vi "User Console.vi"(8 "error in":errorcluster) -> (0 "error out":errorcluster)   [LabVIEW 2025, in "Simulated Console.lvlib"]
doc: "This is the top level of the simulated console module (a free running module of the ATM simulator). \n\nIt is closed using a user event or a local Stop button. It communicates with the other modules using a\nqueue based API which has comms modules that can be swapped if required."
uses:
  Simulated Console.lvlib
  User Events/Controls/UE Abort Action.ctl
  Private Controls/Module Action.ctl
  Private Controls/Module Data Cluster.ctl
  Error Handler/Error Handler.lvlib
  Controller/Contoller.lvlib
  Display/Display Console/Display Console.lvlib
  Private Controls/keypad.ctl
panel:
  in  "Transactions":T1
  in  "Keypad":T2
  in  "Card Reader":bool
  # "[Covers: UI1]"
  # "[Covers: UI2]"
  # "[Covers: UI2A]"
  # "[Covers: UI2B]"
  # "[Covers: UI2C]"
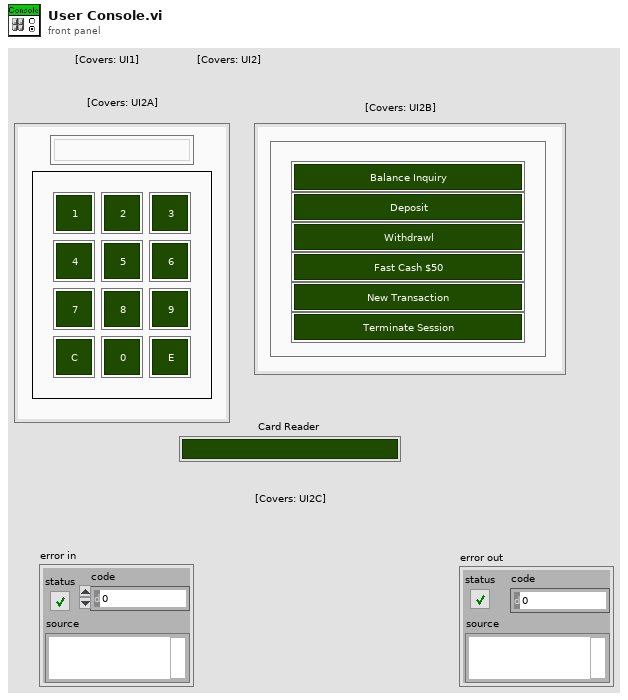
[diagram p1: front panel]
types:
  T1 = cluster{"xaction":bool, "xaction 2":bool, "xaction 3":bool, "xaction 4":bool, "xaction 5":bool, "xaction 6":bool}
  T2 = typedef "Simulated Console.lvlib/keypad.ctl" = cluster{"Key":bool, "Key 2":bool, "Key 3":bool, "Key 4":bool, "Key 5":bool, "Key 6":bool, "Key 7":bool, "Key 8":bool, "Key 9":bool, "Key 10":bool, "Key 11":bool, "Key 12":bool, "Knumber":string}
  T3 = typedef "Simulated Console.lvlib/Module Data Cluster.ctl" = cluster{"Data":variant, "Action":T4}
  T4 = typedef "Simulated Console.lvlib/Module Action.ctl" = enum16{"Error", "Init", "Card", "CancelTransaction", "NewTransaction", "Transaction", "Keypad", "Idle"}
  T5 = typedef "UE Abort Action.ctl" = enum16{"Destroy", "Get", "Create"}
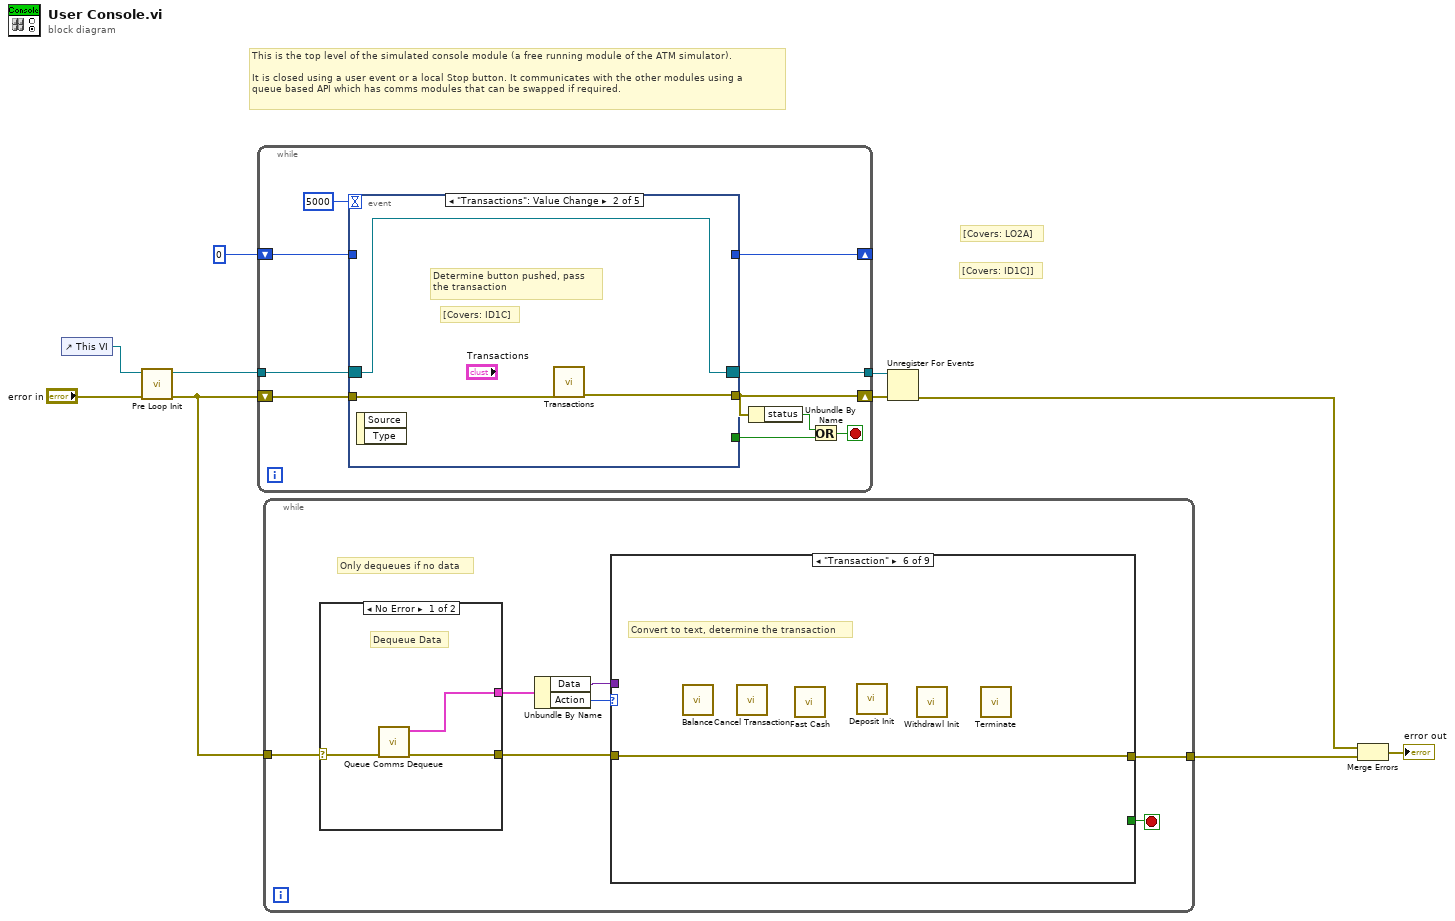
[diagram p0: block diagram]
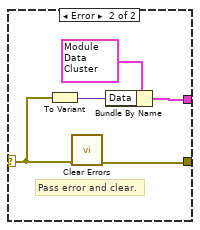
[diagram p2: hidden frame]
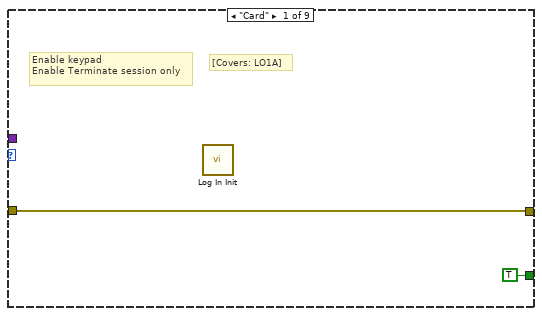
[diagram p3: hidden frame]
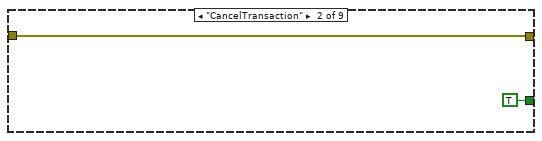
[diagram p4: hidden frame]
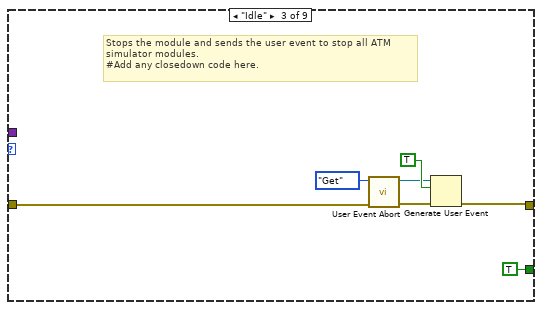
[diagram p5: hidden frame]
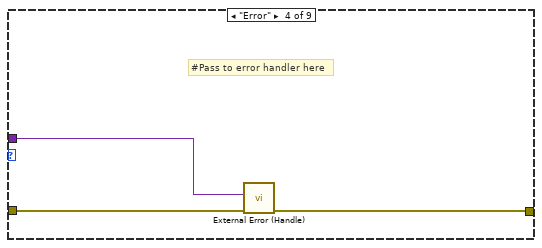
[diagram p6: hidden frame]
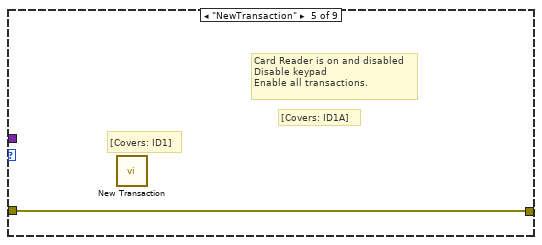
[diagram p7: hidden frame]
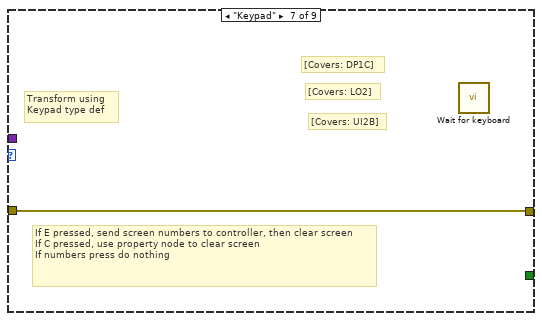
[diagram p8: hidden frame]
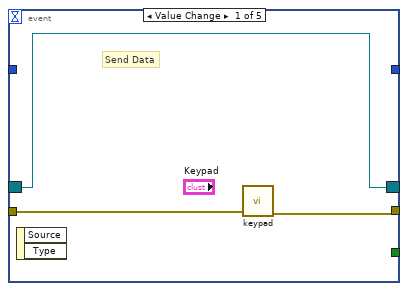
[diagram p11: hidden frame]
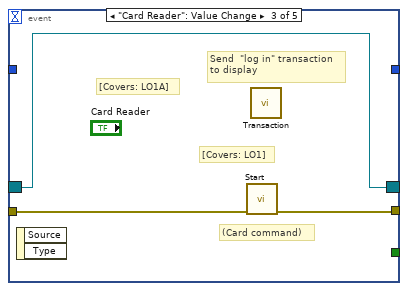
[diagram p12: hidden frame]
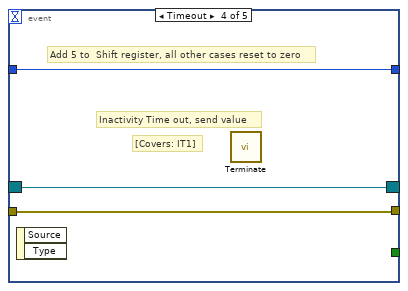
[diagram p13: hidden frame]
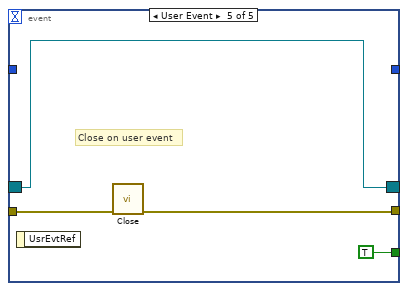
[diagram p14: hidden frame]
diagram:
  # "[Covers: ID1C]]"
  # "[Covers: LO2A]"
  # "This is the top level of the simulated console module (a free running module of the ATM simulator). \n\nIt is closed using a user event or a local Stop button. It communicates with the other modules using a\nqueue based API which has comms modules that can be swapped if required."
  n1 = control-ref of="This VI"() -> (w10:refnum<vi>)
  n2 = call "Pre Loop Init.vi"("error in"="error in", "Ref In"=w10) -> ("error out"=w5:errorcluster, "Event Registration Refnum"=w8:refnum<event-registration>)  [unwired: 8 in]
  n3 = while {
    shift-right: [w17] -> w7
    shift-left: w5 -> [w20]
    tunnel: w8 -> [w15]
    tunnel: [w14] -> w6
    shift-right: [w11] -> _
    shift-left: 0 -> [w12]
    stop <- w18 stop-if-true
    n4 = event shown="[1] \"Transactions\": Value Change" {
      selector: w15 -> [w23 w26 w29 w31 w36]
      dyn-events: [w23 w26 w29 w31 w36] -> w14
      timeout: 5000 -> [_ _ _ _ _]
      tunnel: w20 -> [w22 w25 w28 w32 w35]
      tunnel: [w21 w24 w27 w32 w34] -> w17
      tunnel: [_ _ _ _ TRUE ("stop")] -> w19
      tunnel: w12 -> [_ _ _ w30 _]
      tunnel: [_ _ _ w30 _] -> w11
      event Value Change {
        # "Send Data"
        n5 = event-data() -> ()  [unwired: 1 in, 2 out]
        n6 = call "keypad.vi"("error in"=w22) -> ("error out"=w21:errorcluster)  [unwired: 10 in]
      }
      event "Transactions": Value Change {
        # "[Covers: ID1C]"
        # "Determine button pushed, pass \nthe transaction"
        n7 = event-data() -> ()  [unwired: 1 in, 2 out]
        n8 = call "Transactions.vi"("error in"=w25) -> ("error out"=w24:errorcluster)  [unwired: 10 in]
      }
      event "Card Reader": Value Change {
        # "Send  \"log in\" transaction\nto display"
        # "[Covers: LO1A]"
        # "(Card command)"
        # "[Covers: LO1]"
        n9 = event-data() -> ()  [unwired: 1 in, 2 out]
        n10 = call "Start.vi"("error in"=w28) -> ("error out"=w27:errorcluster)  [unwired: 10 in]
        n11 = call "Transaction.vi"() -> ()  [unwired: 11 in, 1 out]
      }
      event Timeout {
        # "Add 5 to  Shift register, all other cases reset to zero"
        # "[Covers: IT1]"
        # "Inactivity Time out, send value"
        n12 = event-data() -> ()  [unwired: 1 in, 2 out]
        n13 = call "Terminate.vi"() -> ()  [unwired: 11 in, 1 out]
      }
      event User Event {
        # "Close on user event"
        n14 = event-data() -> ()  [unwired: 1 in, 1 out]
        n15 = call "Close.vi"("error in"=w35) -> ("error out"=w34:errorcluster)  [unwired: 10 in]
      }
    }
    n16 = Unbundle By Name(w17) -> ("status"=w16:bool)
    n17 = Or(x=w16, y=w19) -> (x .or. y?=w18:bool)
  }
  n18 = while {
    tunnel: w5 -> [w42]
    tunnel: [w37] -> w3
    stop <- w43 stop-if-true
    # "Only dequeues if no data"
    n19 = case shown="No Error" w42 {
      selector: w42 -> [w45 w48]
      tunnel: [w46 w47] -> w40
      tunnel: [w44 w49] -> w41
      frame No Error {
        # "Dequeue Data"
        n20 = call "Queue Comms Dequeue.vi"("error in"=w45) -> ("error out"=w46:errorcluster, "Data Out"=w44:T3)  [unwired: 9 in]
      }
      frame Error {
        # "Pass error and clear."
        n21 = To Variant(anything=w48) -> (Variant=w50:variant)
        n22 = call <vilib>:"Clear Errors.vi"("error in (no error)"=w48) -> ("error out"=w47:errorcluster)  [unwired: 5 in, 1 out]
        n23 = Bundle By Name(cluster=T3 {"Data"=variant, "Action"=enum."Card"} ("Cluster"), "Data"=w50) -> (w49:T3)
      }
    }
    n24 = Unbundle By Name(w41) -> ("Data"=w38:variant, "Action"=w39:T4)
    n25 = case shown="\"Transaction\"" w39 {
      tunnel: [TRUE TRUE TRUE _ _ _ _ _ _] -> w43
      tunnel: w40 -> [w52 w54 w57 w65 w66 w67 w68 w69 w70]
      tunnel: w38 -> [_ _ _ w63 _ _ _ _ _]
      tunnel: [w52 w54 w56 w64 w66 w67 w68 w69 w70] -> w37
      frame "Card" {
        # "[Covers: LO1A]"
        # "Enable keypad\nEnable Terminate session only"
        n26 = call "Log In Init.vi"() -> ()  [unwired: 11 in, 1 out]
      }
      frame "CancelTransaction" {
      }
      frame "Idle" {
        # "Stops the module and sends the user event to stop all ATM\nsimulator modules. \n#Add any closedown code here."
        n27 = call "User Event Abort.vi"("error in"=w57, "Action"=UE_Abort_Action."Get") -> ("error out"=w59:errorcluster, "user event out"=w60:refnum<user-event>)  [unwired: 8 in]
        n28 = Generate User Event(user event=w60, event data cluster=TRUE ("event data"), error in=w59) -> (error out=w56:errorcluster)  [unwired: 1 in, 1 out]
      }
      frame "Error" {
        # "#Pass to error handler here"
        n29 = call "External Error (Handle).vi"("error in"=w65, "Data"=w63) -> ("error out"=w64:errorcluster)  [unwired: 9 in]
      }
      frame "NewTransaction" {
        # "[Covers: ID1A]"
        # "Card Reader is on and disabled\nDisable keypad\nEnable all transactions."
        # "[Covers: ID1]"
        n30 = call "New Transaction.vi"() -> ()  [unwired: 11 in, 1 out]
      }
      frame "Transaction" {
        # "Convert to text, determine the transaction"
        n31 = call "Balance.vi"() -> ()  [unwired: 11 in, 1 out]
        n32 = call "Cancel Transaction.vi"() -> ()  [unwired: 11 in, 1 out]
        n33 = call "Fast Cash.vi"() -> ()  [unwired: 11 in, 1 out]
        n34 = call "Deposit Init.vi"() -> ()  [unwired: 11 in, 1 out]
        n35 = call "Withdrawl Init.vi"() -> ()  [unwired: 11 in, 1 out]
        n36 = call "Terminate.vi"() -> ()  [unwired: 11 in, 1 out]
      }
      frame "Keypad" {
        # "[Covers: DP1C]"
        # "[Covers: LO2]"
        # "[Covers: UI2B]"
        # "If E pressed, send screen numbers to controller, then clear screen\nIf C pressed, use property node to clear screen\nIf numbers press do nothing"
        # "Transform using \nKeypad type def"
        n37 = call "Wait for keyboard.vi"() -> ()  [unwired: 11 in, 1 out]
      }
      frame "Init", Default {
        # "Enable Card Reader\nDisable all others"
        # "[Covers: IS1]"
      }
      frame "Idle" {
      }
    }
  }
  n38 = Unregister For Events(event registration refnum=w6, error in=w7) -> (error out=w2:errorcluster)
  n39 = Merge Errors(w2, w3) -> (→"error out":errorcluster)
